vi "PRelu.vi"(1 "a":dbl=0.01 min=0.01 step=0.01, 3 "Z":dbl) -> (0 "PRelu(Z)":dbl)   [LabVIEW 2020]
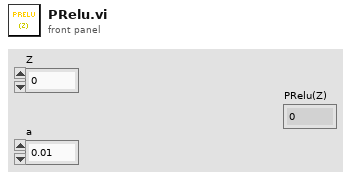
[diagram p1: front panel]
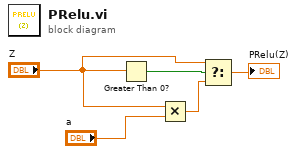
[diagram p0: block diagram]
diagram:
  n1 = Greater Than 0?(x="Z") -> (x > 0?=w4:bool)
  n2 = Multiply(x="Z", y="a") -> (x*y=w3:dbl)
  n3 = Select(t="Z", s=w4, f=w3) -> (s? t:f=→"PRelu(Z)":dbl)
